vi "writeToBinary_bu.vi"(1 "Skip Processing":bool, 2 "Delay A":dbl format="%#_13g", 3 "wavenumber vector":dbl[](array[numeric]), 4 "FFTW3 arrays":T3, 5 "OCT settings":T4, 6 "Buffer in":dbl[][](array[numeric]), 7 "Scan":refnum<class "Scan.lvclass">, 8 "error in":errorcluster, 9 "Progress":refnum<vi>, 10 "Updated camera":T6, 11 "File control":T5={"Subject ID"="", "Eye"=FALSE, "Output Path"=path "E:/test", "String"="", "String 2"=""}) -> (0 "error out":errorcluster)   [LabVIEW 2017]
uses:
  <vilib>/vision/Image Controls.llb/IMAQ Image.ctl
  classes/HardwareObjects/Spectrometer/Spectrometer.lvclass
  classes/HardwareObjects/Camera/Camera.lvclass
  classes/HardwareObjects/DAQ/DAQ.lvclass
  classes/HardwareObjects/Galvonometer/Galvonometer.lvclass
  classes/HardwareObjects/PC/PC.lvclass
  classes/SoftwareObjects/ConfigProc/ConfigProc.lvclass
  classes/Scans/Scan.lvclass
  <vilib>/Analysis/NI_AALBase.lvlib
panel:
  out "hist(FFT)":T1(graph)
  out "size(s)":i32
  out "Post-FFT":dbl[][](graph)
  out "Raw camera output":T2(plugin-control)
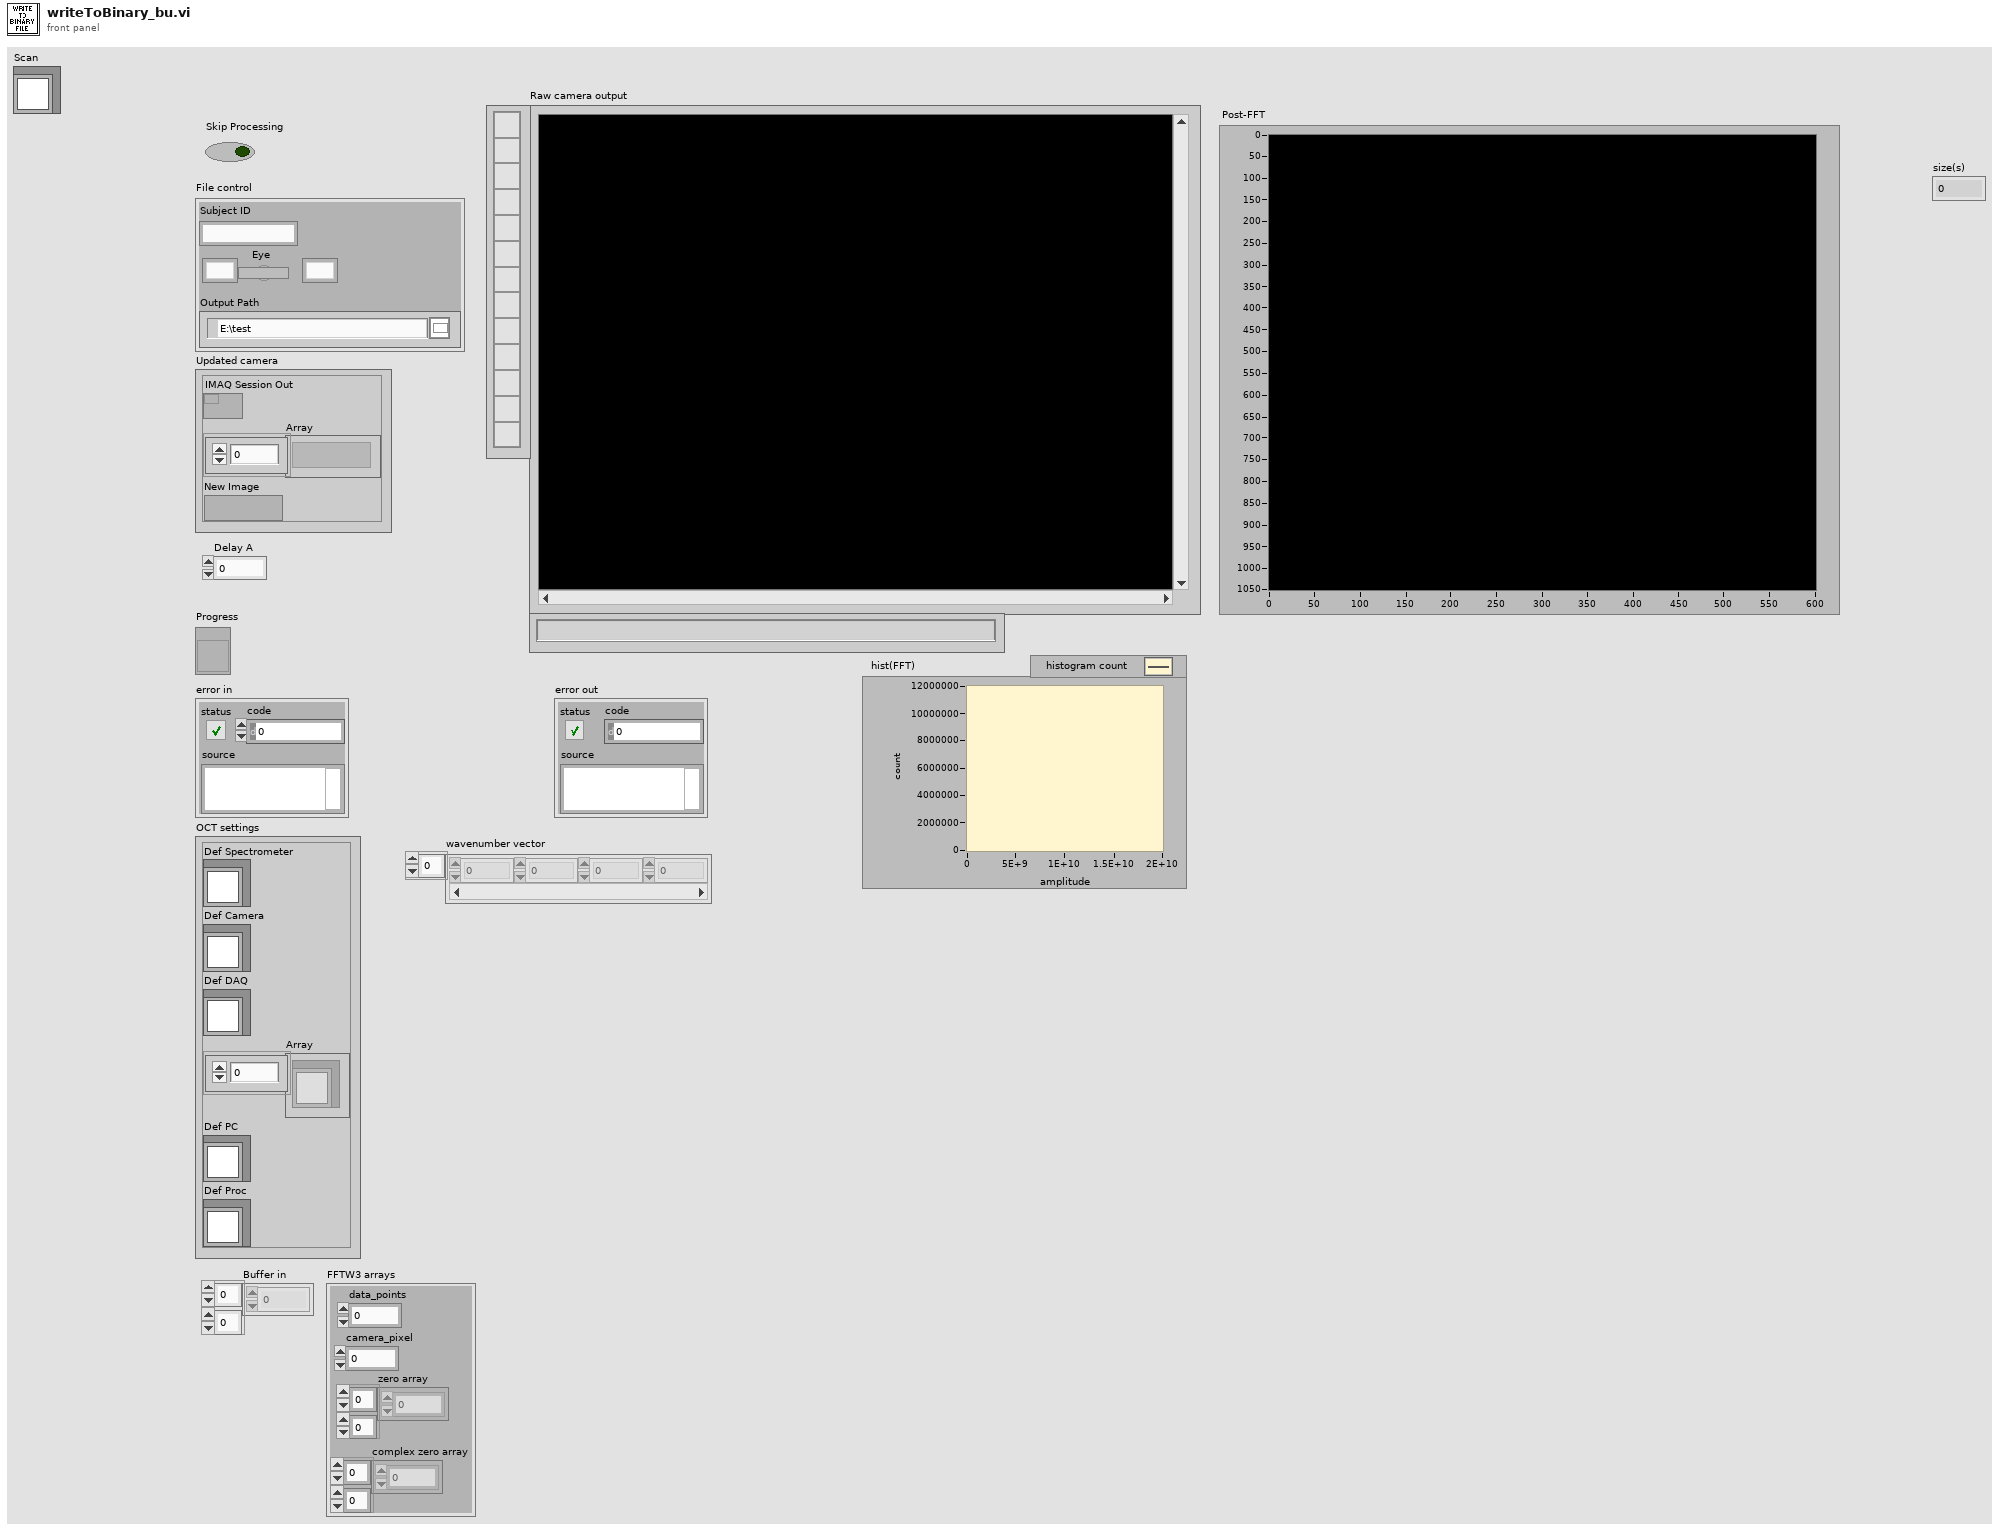
[diagram p1: front panel]
types:
  T1 = cluster{"X Values":dbl[], "Histogram: h(x)":i32[]}
  T2 = typedef "IMAQ Image.ctl" = refnum<image>
  T3 = cluster{"data_points":i32, "camera_pixel":i32, "zero array":dbl[][], "complex zero array":dbl[][]}
  T4 = cluster{"Def Spectrometer":refnum<class "Spectrometer.lvclass">, "Def Camera":refnum<class "Camera.lvclass">, "Def DAQ":refnum<class "DAQ.lvclass">, "Array":refnum<class "Galvonometer.lvclass">[], "Def PC":refnum<class "PC.lvclass">, "Def Proc":refnum<class "ConfigProc.lvclass">}
  T5 = cluster{"Subject ID":string, "Eye":bool, "Output Path":path, "String":string, "String 2":string}
  T6 = cluster{"IMAQ Session Out":refnum<k11>, "Array":T2[], "New Image":T2}
  T7 = enum16{"big-endian, network order", "native, host order", "little-endian"}
  T8 = enum16{"open", "replace", "create", "open or create", "replace or create", "replace or create with confirmation"}
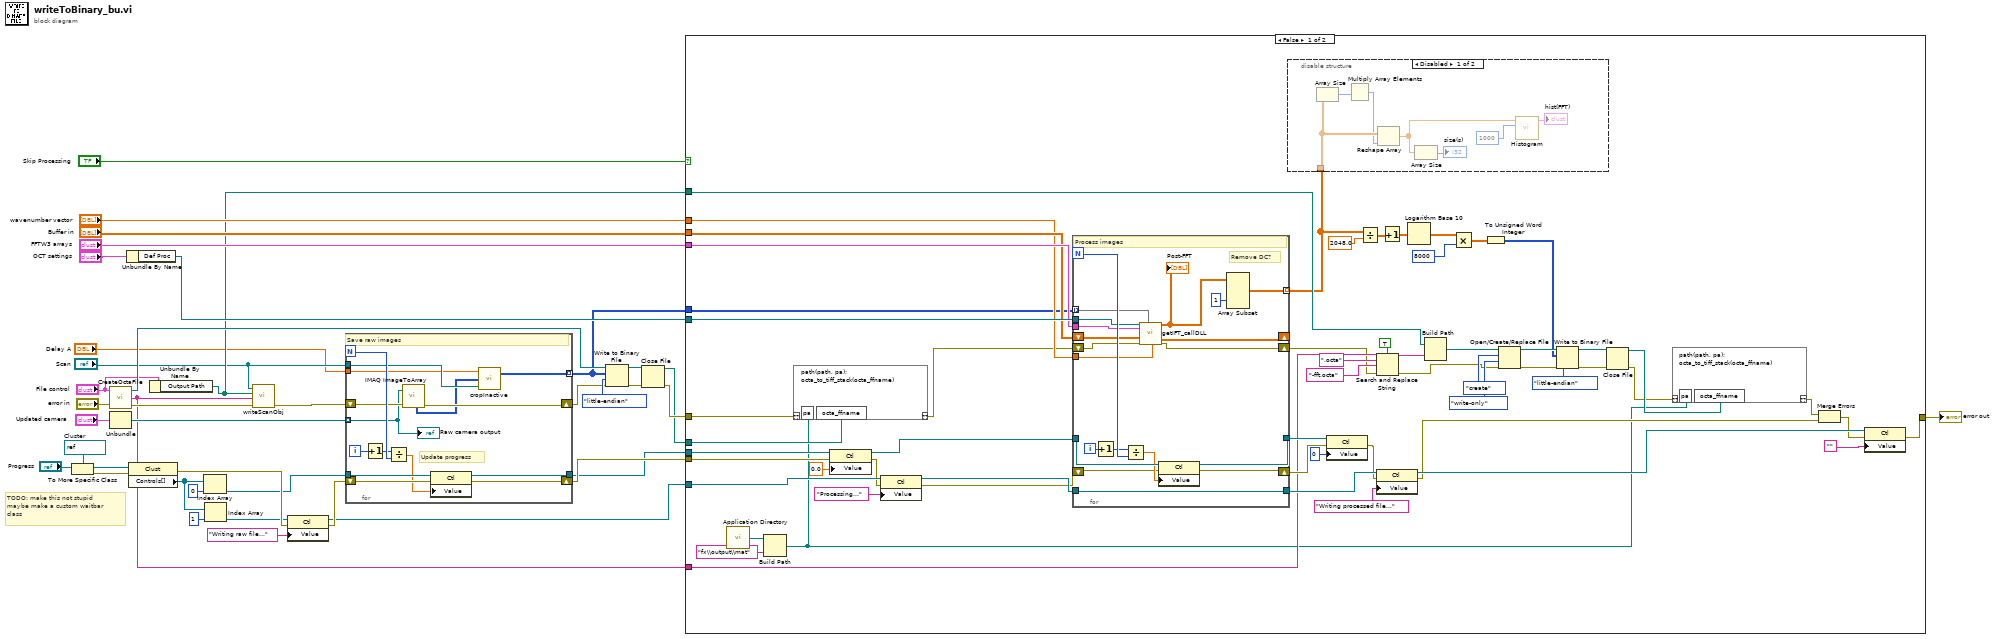
[diagram p0: block diagram]
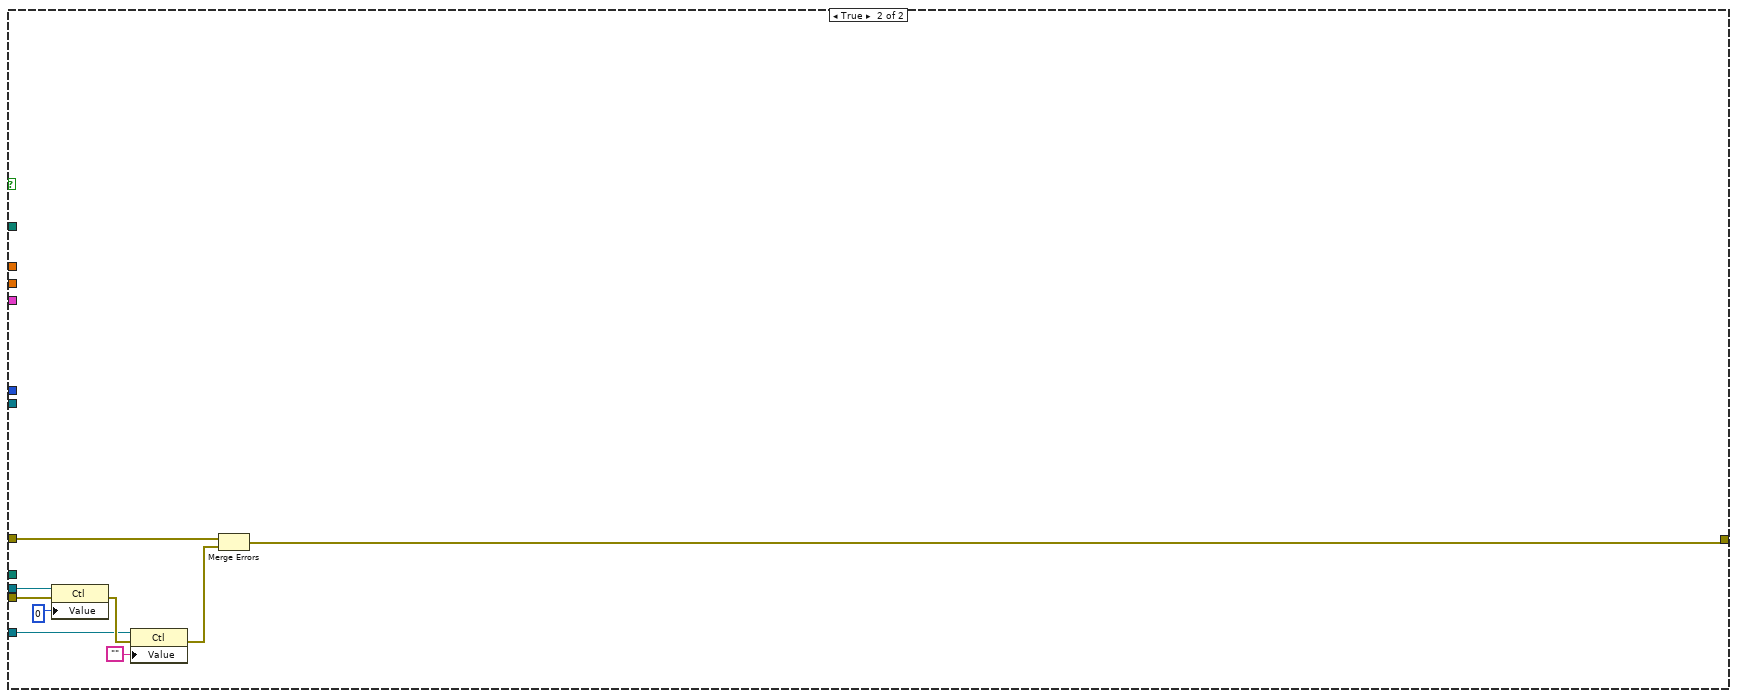
[diagram p3: hidden frame]
diagram:
  w25 = refnum<vi> refnum  # Cluster
  # "TODO: make this not stupid\nmaybe make a custom waitbar\nclass"
  n1 = To More Specific Class(target class=w25, reference="Progress") -> (specific class reference=w24:refnum<vi>, error out=w20:errorcluster)  [unwired: 1 in]
  n2 = call "CreateOctaFile.vi"("error in"="error in", "File control"="File control") -> ("error out"=w12:errorcluster, "OCT filename out"=w8:string, "OCTA refnum out"=w30:refnum<file>)  [unwired: 1 in]
  n3 = Unbundle("Updated camera") -> ("Array"=w36:T2[])  [unwired: 2 out]
  n4 = Unbundle By Name("OCT settings") -> ("Def Proc"=w16:refnum<class "ConfigProc.lvclass">)
  n5 = property class="Clust"(reference=w24, error in=w20) -> (error out=w39:errorcluster, "Controls[]"=w27:refnum<vi>[])  [unwired: 1 out]
  n6 = Unbundle By Name("File control") -> ("Output Path"=w6:path)
  n7 = Index Array(array=w27, index=0) -> (element=w28:refnum<vi>)
  n8 = Index Array(array=w27, index=1) -> (element=w22:refnum<vi>)
  n9 = call "writeScanObj.vi"("error in"=w12, "OCT filename in"=w8, "Output Path"=w6, "Scan"="Scan") -> ("error out"=w11:errorcluster)  [unwired: 3 in]
  n10 = property class="Ctl"(reference=w22, error in=w39, "Value"="Writing raw file...") -> (reference out=w18:refnum<vi>, error out=w19:errorcluster)
  n11 = for {
    N -> [w55]
    tunnel: w36 -> [w45] mode=indexing
    shift-right: [w54] -> w32
    shift-left: w11 -> [w53]
    tunnel: w28 -> [w51]
    shift-right: [w50] -> w40
    shift-left: w19 -> [w49]
    tunnel: [w48] -> w37
    tunnel: [w42] -> w4 mode=indexing
    tunnel: "Scan" -> [w44]
    tunnel: "Delay A" -> [w41]
    i -> [w46]
    # "Update progress"
    # "Save raw images"
    n12 = Increment(x=w46) -> (x+1=w52:i32)
    n13 = Divide(x=w52, y=w55) -> (x/y=w47:dbl)
    n14 = call "IMAQ ImageToArray"("error in (no error)"=w53, "Image"=w45) -> ("Image Pixels (U16)"=w43:u16[][], "error out"=w54:errorcluster)  [unwired: 2 in, 3 out]
    n15 = property class="Ctl"(reference=w51, error in=w49, "Value"=w47) -> (reference out=w48:refnum<vi>, error out=w50:errorcluster)
    n16 = call "cropInactive.vi"("Scan in"=w44, "Whole camera frame"=w43, "Delay A"=w41) -> ("Cropped camera frame"=w42:u16[][])  [unwired: 1 in]
    "Raw camera output" <- w45
  }
  n17 = Write to Binary File(file (use dialog)=w30, data=w4, error in=w32, 9:T7."little-endian" ("byte order (0:big-endian, network order)")) -> (refnum out=w33:refnum<file>, error out=w34:errorcluster)  [unwired: 2 in, 1 out]
  n18 = Close File(refnum=w33, error in=w34) -> (path=w7:path, error out=w9:errorcluster)
  n19 = case shown="False" "Skip Processing" {
    tunnel: w40 -> [w113 w148]
    tunnel: w37 -> [w112 w149]
    tunnel: w18 -> [w110 w145]
    tunnel: w16 -> [w108 _]
    tunnel: "FFTW3 arrays" -> [w107 _]
    tunnel: "Buffer in" -> [w106 _]
    tunnel: "wavenumber vector" -> [w105 _]
    tunnel: w9 -> [w96 w142]
    tunnel: w8 -> [w95 _]
    tunnel: w7 -> [w77 _]
    tunnel: w6 -> [w76 _]
    tunnel: [w68 w141] -> w5
    tunnel: w4 -> [w67 _]
    frame False {
      n20 = call <vilib>:"Application Directory.vi"() -> ("Application Directory"=w58:path)
      n21 = Build Path(base path=w58, name or relative path="fx\\output\\mat") -> (appended path=w56:path)
      n22 = script code="path(path, pa);\nocta_to_tiff_stack(octa_ffname)"("??"=w96, "pa"=w56, "octa_ffname"=w77) -> ("??"=w92:errorcluster)
      n23 = property class="Ctl"(reference=w112, error in=w113, "Value"=sgl 0.0) -> (reference out=w104:refnum<vi>, error out=w102:errorcluster)
      n24 = property class="Ctl"(reference=w110, error in=w102, "Value"="Processing...") -> (reference out=w103:refnum<vi>, error out=w91:errorcluster)
      n25 = for {
        N -> [w140]
        tunnel: w108 -> [w139]
        tunnel: w107 -> [w137]
        shift-right: [w133] -> _
        shift-left: w106 -> [w136]
        tunnel: w105 -> [w135]
        shift-right: [w134] -> w90
        shift-left: w92 -> [w138]
        tunnel: w104 -> [w132]
        tunnel: w103 -> [w131]
        tunnel: [w131] -> w98
        shift-right: [w126] -> w100
        shift-left: w91 -> [w127]
        tunnel: [w125] -> w101
        tunnel: w67 -> [w121] mode=indexing
        tunnel: [w122] -> w60 mode=indexing
        i -> [w130]
        # "Remove DC?"
        # "Process images"
        n26 = Increment(x=w130) -> (x+1=w129:i32)
        n27 = Divide(x=w129, y=w140) -> (x/y=w128:dbl)
        n28 = call "getIFT_callDLL.vi"("Processing Configuration"=w139, "FFTW3 arrays"=w137, "Buffer in"=w136, "error in (no error)"=w138, "Interferogram"=w121, "Spectrum calibration"=w135) -> ("Depth Profile"=w123:dbl[][], "Buffer out"=w133:dbl[][], "error in (no error) 2"=w134:errorcluster)  [unwired: 10 in, 1 out]
        "Post-FFT" <- w123
        n29 = property class="Ctl"(reference=w132, error in=w127, "Value"=w128) -> (reference out=w125:refnum<vi>, error out=w126:errorcluster)
        n30 = Array Subset(array=w123, index (col)=1 ("index")) -> (w122:dbl[][])  [unwired: 3 in]
      }
      n31 = disable-structure shown="Disabled" {
        disable-tunnel: w60 -> [w116 _]
        frame Disabled {
          n32 = Array Size(array=w116) -> (size(s)=w115:i32[])
          n33 = Multiply Array Elements(1:w115) -> (0:w114:i32)
          n34 = Reshape Array(w116, w114) -> (w120:dbl[])
          n35 = Array Size(array=w120) -> (size(s)=→"size(s)":i32)
          n36 = call <vilib>:"Histogram.vi"("intervals"=1000, "X"=w120) -> ("Histogram Graph"=→"hist(FFT)":T1)  [unwired: 6 in, 3 out]
        }
        frame Enabled {
        }
      }
      n37 = property class="Ctl"(reference=w101, error in=w100, "Value"=0) -> (error out=w97:errorcluster)  [unwired: 1 out]
      n38 = Divide(x=w60, y=2048.0) -> (x/y=w65:dbl[][][])
      n39 = Search and Replace String(case sensitive?=TRUE ("ignore case? (F)"), input string=w95, search string=".octa" ("substring (\"\")"), replace string="-fft.octa" ("replace string (\"\")"), error in=w90) -> (result string=w88:string, error out=w84:errorcluster)  [unwired: 3 in, 2 out]
      n40 = property class="Ctl"(reference=w98, error in=w97, "Value"="Writing processed file...") -> (reference out=w72:refnum<vi>, error out=w70:errorcluster)
      n41 = Increment(x=w65) -> (x+1=w64:dbl[][][])
      n42 = Logarithm Base 10(1:w64) -> (0:w63:dbl[][][])
      n43 = Build Path(base path=w76, name or relative path=w88) -> (appended path=w87:path)
      n44 = Multiply(x=w63, y=8000) -> (x*y=w61:dbl[][][])
      n45 = To Unsigned Word Integer(number=w61) -> (unsigned 16bit integer=w59:u16[][][])
      n46 = Open/Create/Replace File(file path (use dialog)=w87, error in=w84, operation (0:open)=T8."create", access (0:read/write)=enum16{"read/write", "read-only", "write-only"}."write-only") -> (refnum out=w81:refnum<file>, error out=w82:errorcluster)  [unwired: 2 in, 1 out]
      n47 = Write to Binary File(file (use dialog)=w81, data=w59, error in=w82, 9:T7."little-endian" ("byte order (0:big-endian, network order)")) -> (refnum out=w78:refnum<file>, error out=w79:errorcluster)  [unwired: 2 in, 1 out]
      n48 = Close File(refnum=w78, error in=w79) -> (path=w75:path, error out=w74:errorcluster)
      n49 = script code="path(path, pa);\nocta_to_tiff_stack(octa_ffname)"("??"=w74, "pa"=w56, "octa_ffname"=w75) -> ("??"=w73:errorcluster)
      n50 = Merge Errors(w73, w70) -> (w69:errorcluster)
      n51 = property class="Ctl"(reference=w72, error in=w69, "Value"="") -> (error out=w68:errorcluster)  [unwired: 1 out]
    }
    frame True {
      n52 = property class="Ctl"(reference=w149, error in=w148, "Value"=0) -> (error out=w146:errorcluster)  [unwired: 1 out]
      n53 = property class="Ctl"(reference=w145, error in=w146, "Value"="") -> (error out=w143:errorcluster)  [unwired: 1 out]
      n54 = Merge Errors(w142, w143) -> (w141:errorcluster)
    }
  }
  "error out" <- w5
